vi "Threshold_4ch_v00.vi"(6 "MaxMin":T1, 11 "Signals":T12={"PII In 1"={"Lock"=FALSE, "Hold"=FALSE, "P Gain"=0, "P BS"=0, "I Gain"=0, "I BS"=-10, "I2 G"=0, "I2 BS"=-26, "Scan Amp"=0, "Scan Off"=0, "Scan FS"=0, "SFS BS"=0, "I Max value"=10000, "I2 Max value"=10000, "Scope.Offset"=0, "Trigger Direction"=enum."either", "Scan-PII thresh"=0}, "PII In 2"={"Lock"=FALSE, "Hold"=FALSE, "P Gain"=0, "P BS"=0, "I Gain"=0, "I BS"=-10, "I2 G"=0, "I2 BS"=-26, "Scan Amp"=0, "Scan Off"=0, "Scan FS"=0, "SFS BS"=0, "I Max value"=10000, "I2 Max value"=10000, "Scope.Offset"=0, "Trigger Direction"=enum."either", "Scan-PII thresh"=0}, "PII In 3"={"Lock"=FALSE, "Hold"=FALSE, "P Gain"=0, "P BS"=0, "I Gain"=0, "I BS"=-10, "I2 G"=0, "I2 BS"=-26, "Scan Amp"=0, "Scan Off"=0, "Scan FS"=0, "SFS BS"=0, "I Max value"=10000, "I2 Max value"=10000, "Scope.Offset"=0, "Trigger Direction"=enum."either", "Scan-PII thresh"=0}, "Lock Thresh"={"EPR"=2, "HD A"=0, "HD B"=0, "HD C"=0}, "Re-Scan Thresh"={"EPR"=2, "HD A"=0, "HD B"=0, "HD C"=0}, "Safety First"={"lim reset"=FALSE, "no limit"=FALSE, "pos slew rate * dt"=0, "neg slew rate * dt"=-10, "Hold All"=FALSE, "Count(Ticks)"=4294967286}, "Graph Errors"={"EPR"=2, "HD A"=0, "HD B"=0, "HD C"=0}, "PII In 4"={"Lock"=FALSE, "Hold"=FALSE, "P Gain"=0, "P BS"=-10, "I Gain"=0, "I BS"=-10, "I2 G"=0, "I2 BS"=-26, "Scan Amp"=0, "Scan Off"=0, "Scan FS"=0, "SFS BS"=0, "I Max value"=10000, "I2 Max value"=10000, "Scope.Offset"=0, "Trigger Direction"=enum."either", "Scan-PII thresh"=0}}) -> (3 "Control Graph Cluster":T8={"Control EPR"={"Lock"=FALSE, "Hold"=FALSE, "P Gain"=0, "P BS"=-5, "I Gain"=0, "I BS"=-10, "I2 G"=0, "I2 BS"=-26, "Scan Amp"=0, "Scan Off"=0, "Scan FS"=0, "SFS BS"=0, "I Max value"=10000, "I2 Max value"=10000, "Scope.Offset"=0, "Trigger Direction"=enum."either", "Scan-PII thresh"=0}, "Control HD A"={"Lock"=FALSE, "Hold"=FALSE, "P Gain"=0, "P BS"=-5, "I Gain"=0, "I BS"=-10, "I2 G"=0, "I2 BS"=-26, "Scan Amp"=0, "Scan Off"=0, "Scan FS"=0, "SFS BS"=0, "I Max value"=10000, "I2 Max value"=10000, "Scope.Offset"=0, "Trigger Direction"=enum."either", "Scan-PII thresh"=0}, "Control HD B"={"Lock"=FALSE, "Hold"=FALSE, "P Gain"=0, "P BS"=-5, "I Gain"=0, "I BS"=-10, "I2 G"=0, "I2 BS"=-26, "Scan Amp"=0, "Scan Off"=0, "Scan FS"=0, "SFS BS"=0, "I Max value"=10000, "I2 Max value"=10000, "Scope.Offset"=0, "Trigger Direction"=enum."either", "Scan-PII thresh"=0}, "Max"={"Max EPR"=0, "Max HD A"=0, "Max HD B"=0, "Max HD C"=0}, "Min"={"Min EPR"=0, "Min HD A"=0, "Min HD B"=0, "Min HD C"=0}, "Lock Threshold"={"EPR"=0, "HD A"=0, "HD B"=0, "HD C"=0}, "Re-Scan Threshold"={"EPR"=0, "HD A"=0, "HD B"=0, "HD C"=0}, "Lock Point?"={"EPR"=FALSE, "HD A"=FALSE, "HD B"=FALSE, "HD C"=FALSE}, "Re-scan?"={"EPR"=FALSE, "HD A"=FALSE, "HD B"=FALSE, "HD C"=FALSE}, "Lock pressed? (-1)"={"EPR"=FALSE, "HD A"=FALSE, "HD B"=FALSE, "HD C"=FALSE}, "Cavity Errors"={"EPR"=0, "HD A"=0, "HD B"=0, "HD C"=0}, "State (-1)"={"EPR"=enum."Safe", "HD A"=enum."Safe", "HD B"=enum."Safe", "HD C"=enum."Safe"}, "Safety First"={"lim reset"=FALSE, "no limit"=FALSE, "pos slew rate * dt"=0, "neg slew rate * dt"=0, "Hold All"=FALSE, "Count(Ticks)"=0}, "Control HD C"={"Lock"=FALSE, "Hold"=FALSE, "P Gain"=0, "P BS"=-5, "I Gain"=0, "I BS"=-10, "I2 G"=0, "I2 BS"=-26, "Scan Amp"=0, "Scan Off"=0, "Scan FS"=0, "SFS BS"=0, "I Max value"=10000, "I2 Max value"=10000, "Scope.Offset"=0, "Trigger Direction"=enum."either", "Scan-PII thresh"=0}})   [LabVIEW 2013]
doc: "Determines if the relative phase of the two interfering beams are within a range determined by a user-defined threshold. The absolute value of the error signal is used as a monitor."
uses:
  Strict Type Defs/1BS3HD Signals.ctl
  Strict Type Defs/PII individual.ctl
  Strict Type Defs/1BS3HD Lock Thresh.ctl
  Strict Type Defs/Safety First.ctl
  Strict Type Defs/1BS3HD Error Signals.ctl
  Strict Type Defs/1BS3HD Control Cluster.ctl
  Strict Type Defs/1BS3HD Max.ctl
  Strict Type Defs/1BS3HD Min.ctl
  Strict Type Defs/1BS3HD Lock Point.ctl
  Strict Type Defs/1BS3HD State.ctl
  Strict Type Defs/1BS3HD MaxMin.ctl
  Strict Type Defs/1BS3HD Reset MaxMin.ctl
panel:
  in  "Control Cavity Cluster":T8={"Control EPR"={"Lock"=FALSE, "Hold"=FALSE, "P Gain"=0, "P BS"=-5, "I Gain"=0, "I BS"=-10, "I2 G"=0, "I2 BS"=-26, "Scan Amp"=0, "Scan Off"=0, "Scan FS"=0, "SFS BS"=0, "I Max value"=10000, "I2 Max value"=10000, "Scope.Offset"=0, "Trigger Direction"=enum."either", "Scan-PII thresh"=0}, "Control HD A"={"Lock"=FALSE, "Hold"=FALSE, "P Gain"=0, "P BS"=-5, "I Gain"=0, "I BS"=-10, "I2 G"=0, "I2 BS"=-26, "Scan Amp"=0, "Scan Off"=0, "Scan FS"=0, "SFS BS"=0, "I Max value"=10000, "I2 Max value"=10000, "Scope.Offset"=0, "Trigger Direction"=enum."either", "Scan-PII thresh"=0}, "Control HD B"={"Lock"=FALSE, "Hold"=FALSE, "P Gain"=0, "P BS"=-5, "I Gain"=0, "I BS"=-10, "I2 G"=0, "I2 BS"=-26, "Scan Amp"=0, "Scan Off"=0, "Scan FS"=0, "SFS BS"=0, "I Max value"=10000, "I2 Max value"=10000, "Scope.Offset"=0, "Trigger Direction"=enum."either", "Scan-PII thresh"=0}, "Max"={"Max EPR"=0, "Max HD A"=0, "Max HD B"=0, "Max HD C"=0}, "Min"={"Min EPR"=0, "Min HD A"=0, "Min HD B"=0, "Min HD C"=0}, "Lock Threshold"={"EPR"=0, "HD A"=0, "HD B"=0, "HD C"=0}, "Re-Scan Threshold"={"EPR"=0, "HD A"=0, "HD B"=0, "HD C"=0}, "Lock Point?"={"EPR"=FALSE, "HD A"=FALSE, "HD B"=FALSE, "HD C"=FALSE}, "Re-scan?"={"EPR"=FALSE, "HD A"=FALSE, "HD B"=FALSE, "HD C"=FALSE}, "Lock pressed? (-1)"={"EPR"=FALSE, "HD A"=FALSE, "HD B"=FALSE, "HD C"=FALSE}, "Cavity Errors"={"EPR"=0, "HD A"=0, "HD B"=0, "HD C"=0}, "State (-1)"={"EPR"=enum."Safe", "HD A"=enum."Safe", "HD B"=enum."Safe", "HD C"=enum."Safe"}, "Safety First"={"lim reset"=FALSE, "no limit"=FALSE, "pos slew rate * dt"=0, "neg slew rate * dt"=0, "Hold All"=FALSE, "Count(Ticks)"=0}, "Control HD C"={"Lock"=FALSE, "Hold"=FALSE, "P Gain"=0, "P BS"=-5, "I Gain"=0, "I BS"=-10, "I2 G"=0, "I2 BS"=-26, "Scan Amp"=0, "Scan Off"=0, "Scan FS"=0, "SFS BS"=0, "I Max value"=10000, "I2 Max value"=10000, "Scope.Offset"=0, "Trigger Direction"=enum."either", "Scan-PII thresh"=0}}
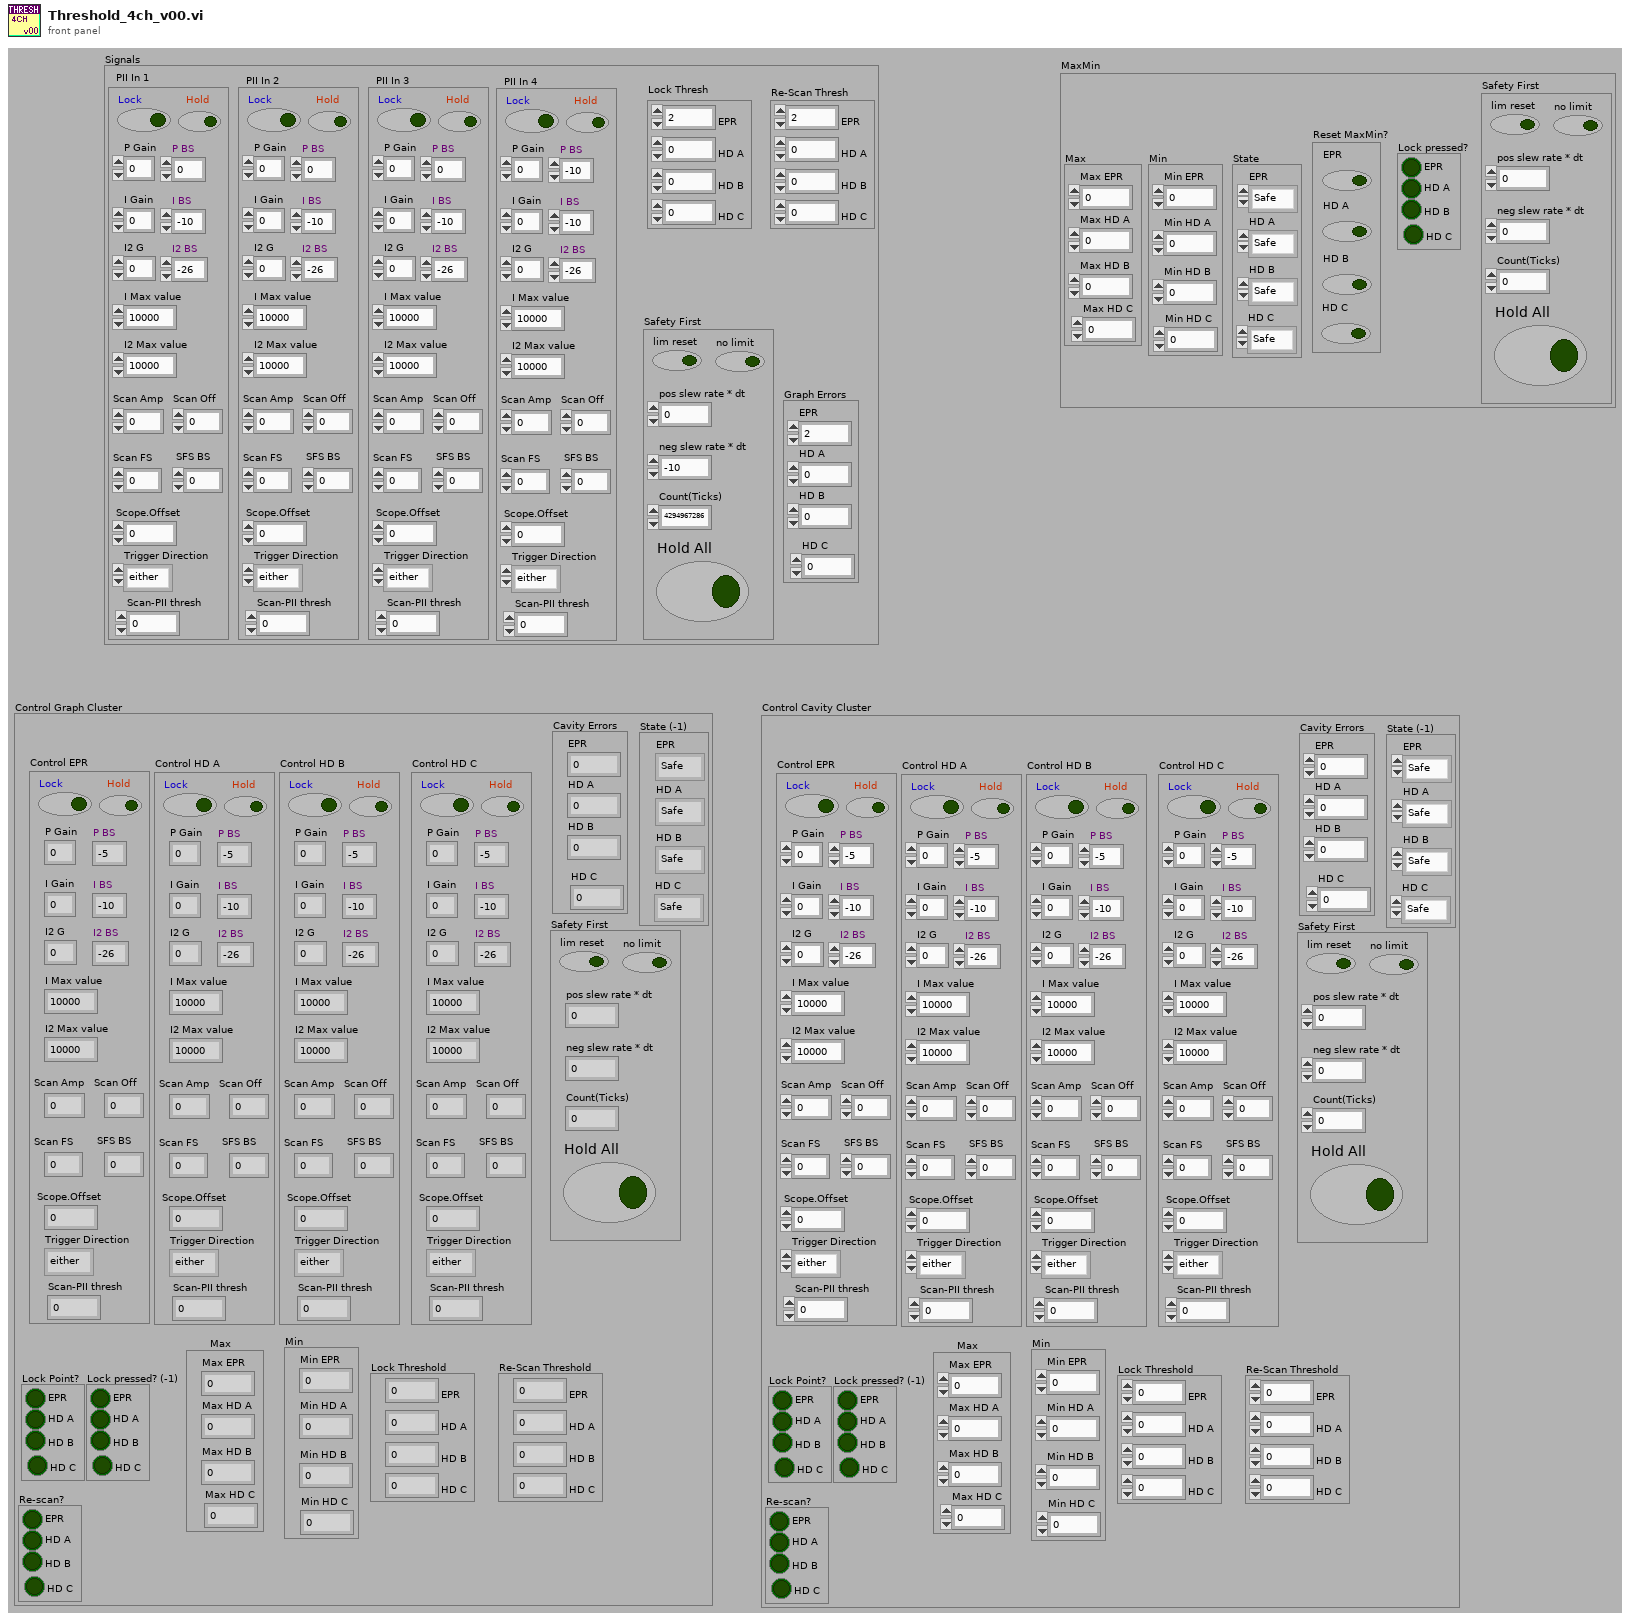
[diagram p1: front panel]
types:
  T1 = typedef "1BS3HD MaxMin.ctl" = cluster{"State":T2, "Reset MaxMin?":T3, "Max":T4, "Min":T5, "Lock pressed?":T6, "Safety First":T7}
  T2 = typedef "1BS3HD State.ctl" = cluster{"EPR":enum16{"Safe", "Hold", "Scan", "Lock"}, "HD A":enum16{"Safe", "Hold", "Scan", "Lock"}, "HD B":enum16{"Safe", "Hold", "Scan", "Lock"}, "HD C":enum16{"Safe", "Hold", "Scan", "Lock"}}
  T3 = typedef "1BS3HD Reset MaxMin.ctl" = cluster{"EPR":bool, "HD A":bool, "HD B":bool, "HD C":bool}
  T4 = typedef "1BS3HD Max.ctl" = cluster{"Max EPR":i16, "Max HD A":i16, "Max HD B":i16, "Max HD C":i16}
  T5 = typedef "1BS3HD Min.ctl" = cluster{"Min EPR":i16, "Min HD A":i16, "Min HD B":i16, "Min HD C":i16}
  T6 = typedef "1BS3HD Lock Point.ctl" = cluster{"EPR":bool, "HD A":bool, "HD B":bool, "HD C":bool}
  T7 = typedef "Safety First.ctl" = cluster{"lim reset":bool, "no limit":bool, "pos slew rate * dt":i16, "neg slew rate * dt":i16, "Hold All":bool, "Count(Ticks)":u32}
  T8 = typedef "1BS3HD Control Cluster.ctl" = cluster{"Control EPR":T9, "Control HD A":T9, "Control HD B":T9, "Max":T4, "Min":T5, "Lock Threshold":T10, "Re-Scan Threshold":T10, "Lock Point?":T6, "Re-scan?":T6, "Lock pressed? (-1)":T6, "Cavity Errors":T11, "State (-1)":T2, "Safety First":T7, "Control HD C":T9}
  T9 = typedef "PII individual.ctl" = cluster{"Lock":bool, "Hold":bool, "P Gain":i32, "P BS":i16, "I Gain":i32, "I BS":i16, "I2 G":i32, "I2 BS":i16, "Scan Amp":i16, "Scan Off":i16, "Scan FS":u16, "SFS BS":i16, "I Max value":i32, "I2 Max value":i32, "Scope.Offset":i16, "Trigger Direction":enum8{"either", "minus-plus", "plus-minus"}, "Scan-PII thresh":i16}
  T10 = typedef "1BS3HD Lock Thresh.ctl" = cluster{"EPR":i16, "HD A":i16, "HD B":i16, "HD C":i16}
  T11 = typedef "1BS3HD Error Signals.ctl" = cluster{"EPR":i16, "HD A":i16, "HD B":i16, "HD C":i16}
  T12 = typedef "1BS3HD Signals.ctl" = cluster{"PII In 1":T9, "PII In 2":T9, "PII In 3":T9, "Lock Thresh":T10, "Re-Scan Thresh":T10, "Safety First":T7, "Graph Errors":T11, "PII In 4":T9}
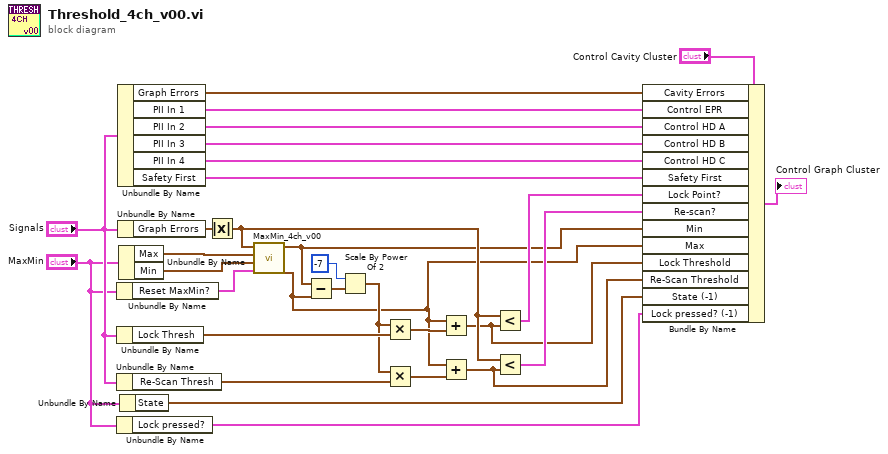
[diagram p0: block diagram]
diagram:
  n1 = Unbundle By Name("MaxMin") -> ("Reset MaxMin?"=w22:T3)
  n2 = Unbundle By Name("Signals") -> ("Lock Thresh"=w18:T10)
  n3 = Unbundle By Name("Signals") -> ("Re-Scan Thresh"=w24:T10)
  n4 = Unbundle By Name("MaxMin") -> ("Lock pressed?"=w3:T6)
  n5 = Unbundle By Name("Signals") -> ("Graph Errors"=w14:T11, "PII In 1"=w13:T9, "PII In 2"=w12:T9, "PII In 3"=w11:T9, "PII In 4"=w1:T9, "Safety First"=w2:T7)
  n6 = Unbundle By Name("Signals") -> ("Graph Errors"=w20:T11)
  n7 = Unbundle By Name("MaxMin") -> ("Max"=w30:T4, "Min"=w29:T5)
  n8 = Unbundle By Name("MaxMin") -> ("State"=w4:T2)
  n9 = Absolute Value(x=w20) -> (abs(x)=w19:T11)
  n10 = call "MaxMin_4ch_v00.vi"("Reset MaxMin?"=w22, "Min (-1)"=w29, "Max (-1)"=w30, "Error Signals"=w19) -> ("Max"=w7:T4, "Min"=w8:T5)  [unwired: 6 in]
  n11 = Subtract(x=w8, y=w7) -> (x-y=w27:T5)
  n12 = Scale By Power Of 2(n=-7, x=w27) -> (x*2^n=w17:T5)
  n13 = Multiply(x=w17, y=w18) -> (x*y=w26:T5)
  n14 = Multiply(x=w17, y=w24) -> (x*y=w25:T5)
  n15 = Add(x=w7, y=w26) -> (x+y=w6:T4)
  n16 = Add(x=w7, y=w25) -> (x+y=w5:T4)
  n17 = Less?(x=w19, y=w6) -> (x < y?=w10:cluster{bool, bool, bool, bool})
  n18 = Less?(x=w19, y=w5) -> (x < y?=w9:cluster{bool, bool, bool, bool})
  n19 = Bundle By Name(cluster="Control Cavity Cluster", "Cavity Errors"=w14, "Control EPR"=w13, "Control HD A"=w12, "Control HD B"=w11, "Control HD C"=w1, "Safety First"=w2, "Lock Point?"=w10, "Re-scan?"=w9, "Min"=w8, "Max"=w7, "Lock Threshold"=w6, "Re-Scan Threshold"=w5, "State (-1)"=w4, "Lock pressed? (-1)"=w3) -> (→"Control Graph Cluster":T8)
